vi "rad_FilterTargets.vi"(8 "error in (no error)":errorcluster, 10 "Target Types":string[](array[string]), 11 "Targets Information":T1[](array[typedef]) {"Primary NIC"."IP Address Request Mode" items=["Static"=1, "DHCP/Link-Local"=2, "Link-Local Only"=4, "DHCP Only"=8]}) -> (0 "error out":errorcluster, 1 "Filtered Targets":i32[](array[numeric]), 3 "Targets Information":T1[](array[typedef]) {"Primary NIC"."IP Address Request Mode" items=["Static"=1, "DHCP/Link-Local"=2, "Link-Local Only"=4, "DHCP Only"=8]})   [LabVIEW 2020]
uses:
  Target Information.ctl
  subVIs/Targets/TypeDefs/rad_Target Network Settings.ctl
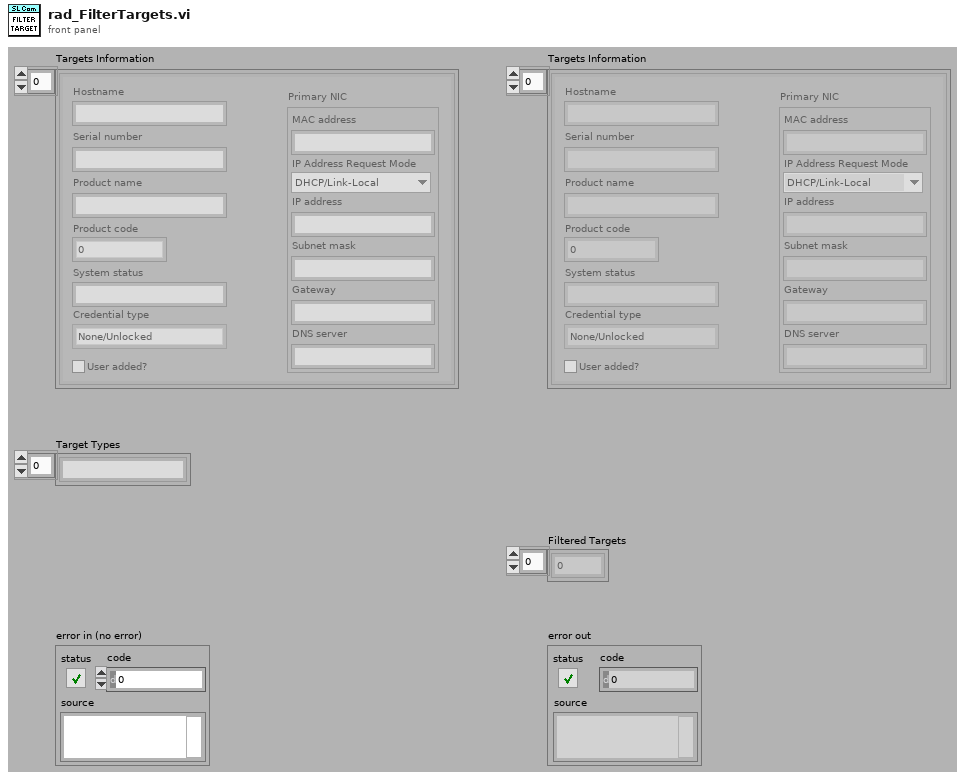
[diagram p1: front panel]
types:
  T1 = typedef "Target Information.ctl" = cluster{"Hostname":string, "Serial number":string, "Product name":string, "Product code":i32, "System status":string, "Credential type":enum16{"None/Unlocked", "FTP Password", "NIAuth Credentials"}, "User added?":bool, "Primary NIC":T2}
  T2 = typedef "rad_Target Network Settings.ctl" = cluster{"MAC address":string, "IP Address Request Mode":i32, "IP address":string, "Subnet mask":string, "Gateway":string, "DNS server":string}
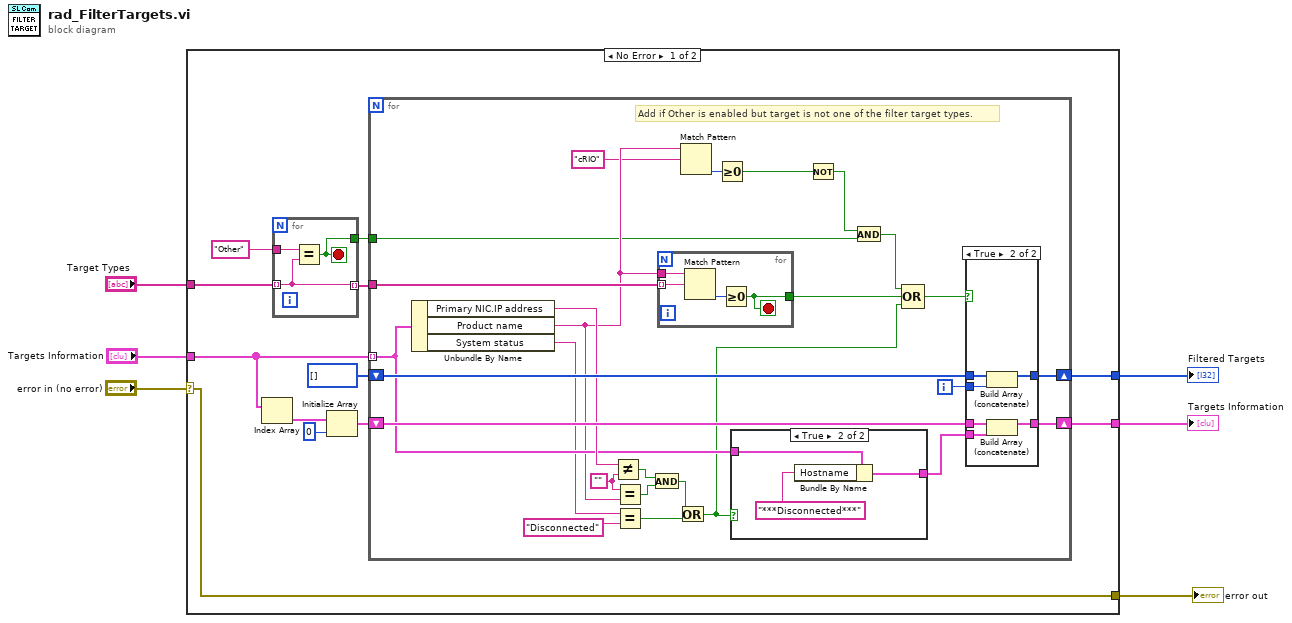
[diagram p0: block diagram]
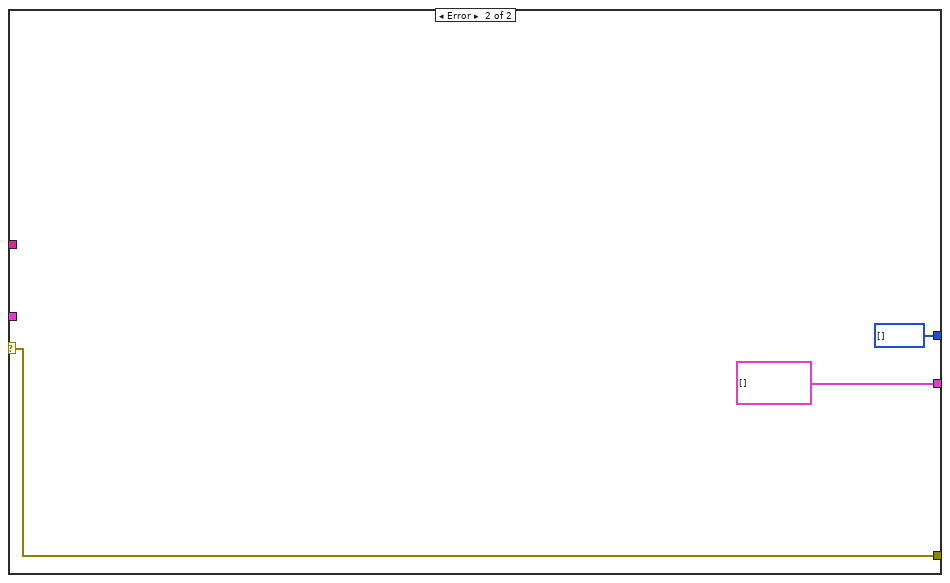
[diagram p4: hidden frame]
diagram:
  n1 = case shown="No Error" "error in (no error)" {
    selector: "error in (no error)" -> [w7 w66]
    tunnel: "Targets Information" -> [w15 _]
    tunnel: [w14 T1[] []] -> w5
    tunnel: [w12 i32[] []] -> w4
    tunnel: "Target Types" -> [w11 _]
    tunnel: [w7 w66] -> w1
    frame No Error {
      n2 = Index Array(array=w15) -> (element=w17:T1)  [unwired: 1 in]
      n3 = for {
        tunnel: w11 -> [w20] mode=indexing
        tunnel: [w20] -> w10 mode=indexing
        tunnel: "Other" ("y") -> [w19]
        tunnel: [w21] -> w8
        stop <- w21 stop-if-true
        n4 = Equal?(x=w19, y=w20) -> (x = y?=w21:bool)
      }
      n5 = Initialize Array(w17, 0 ("dimension size")) -> (w16:T1[])
      n6 = for {
        shift-right: [w46] -> w14
        shift-left: w16 -> [w47]
        tunnel: w15 -> [w36] mode=indexing
        tunnel: w10 -> [w45]
        shift-right: [w43] -> w12
        shift-left: i32[] [] -> [w42]
        tunnel: w8 -> [w25]
        i -> [w44]
        w40 = ""
        # "Add if Other is enabled but target is not one of the filter target types."
        n7 = Unbundle By Name(w36) -> ("Primary NIC.IP address"=w41:string, "Product name"=w28:string, "System status"=w34:string)
        n8 = Not Equal?(x=w41, y=w40) -> (x != y?=w39:bool)
        n9 = Equal?(x=w40, y=w28) -> (x = y?=w38:bool)
        n10 = Equal?(x=w34, y="Disconnected") -> (x = y?=w31:bool)
        n11 = And(x=w39, y=w38) -> (x .and. y?=w32:bool)
        n12 = for {
          tunnel: w28 -> [w55]
          tunnel: w45 -> [w54] mode=indexing
          tunnel: [w52] -> w29
          stop <- w52 stop-if-true
          n13 = Match Pattern(string=w55, regular expression=w54) -> (offset past match=w53:i32)  [unwired: 4 out]
          n14 = Greater Or Equal To 0?(x=w53) -> (x >= 0?=w52:bool)
        }
        n15 = Or(x=w32, y=w31) -> (x .or. y?=w30:bool)
        n16 = Match Pattern(string=w28, regular expression="cRIO") -> (offset past match=w23:i32)  [unwired: 4 out]
        n17 = Greater Or Equal To 0?(x=w23) -> (x >= 0?=w27:bool)
        n18 = case shown="True" w30 {
          tunnel: w36 -> [w48 w51]
          tunnel: [w48 w49] -> w35
          frame False {
          }
          frame True {
            n19 = Bundle By Name(cluster=w51, "Hostname"="***Disconnected***" ("IP settings.DNS name")) -> (w49:T1)
          }
        }
        n20 = Not(x=w27) -> (.not. x?=w26:bool)
        n21 = And(x=w26, y=w25) -> (x .and. y?=w24:bool)
        n22 = Compound Arithmetic op=OR(w24, w29, w30) -> (w37:bool)
        n23 = case shown="True" w37 {
          tunnel: w47 -> [w57 w63]
          tunnel: [w57 w61] -> w46
          tunnel: w35 -> [_ w62]
          tunnel: w44 -> [_ w60]
          tunnel: [w56 w59] -> w43
          tunnel: w42 -> [w56 w58]
          frame False {
          }
          frame True {
            n24 = Build Array (concatenate)(w58, w60) -> (w59:i32[])
            n25 = Build Array (concatenate)(w63, w62) -> (w61:T1[])
          }
        }
      }
    }
    frame Error {
    }
  }
  "Targets Information" <- w5
  "Filtered Targets" <- w4
  "error out" <- w1
